vi "Open Baseline Image.vi"(8 "error in (no error)":errorcluster) -> (0 "error out":errorcluster, 2 "dup path":path, 3 "Image Out":T1)   [LabVIEW 2011]
uses:
  <vilib>/vision/Image Controls.llb/IMAQ Image.ctl
  <vilib>/Utility/sysdir.llb/System Directory Type.ctl
  DepthSense/IT WORKS SO SUCK IT/DepthSense Global Status.vi
  <vilib>/vision/NI_Vision_Development_Module.lvlib
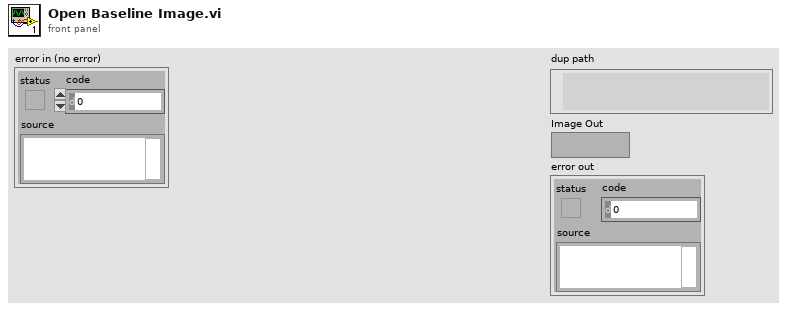
[diagram p1: front panel]
types:
  T1 = typedef "IMAQ Image.ctl" = refnum<image>
  T2 = typedef "System Directory Type.ctl" = i32
  T3 = cluster{"Camera Version":string, "Image Height":i32, "Image Width":i32, "Minimum Framerate":i32, "Maximum Framerate":i32, "Framerate":i32, "Close Mode":bool, "Denoising":bool, "Leakage Algorithm":bool, "Anti-Aliasing":bool, "Camera Status":i32, "API Version":string, "Light Intensity":i32, "Confidence Threshold":u16, "Range":sgl}
  T4 = typedef "Image Type" = u32
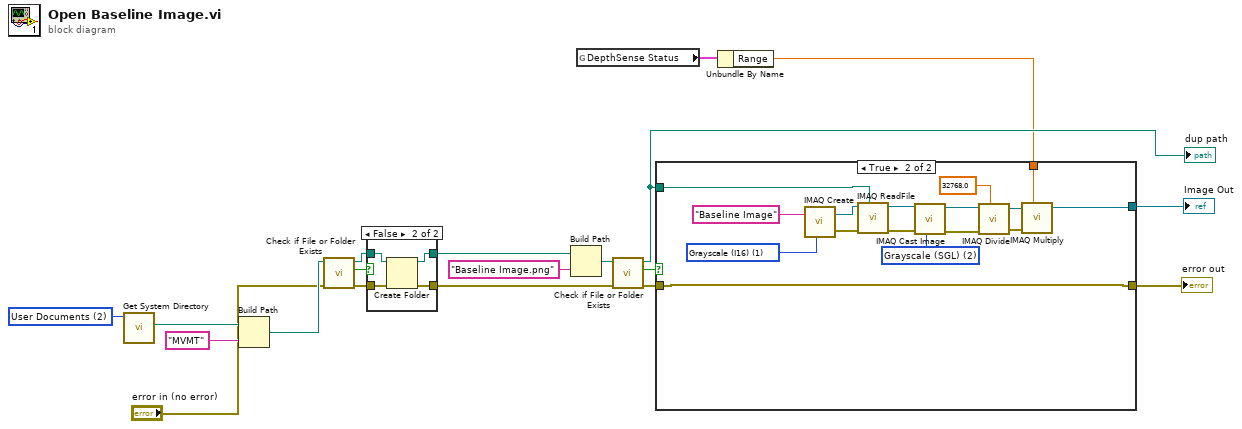
[diagram p0: block diagram]
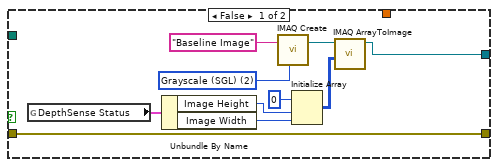
[diagram p2: hidden frame]
diagram:
  w8 = T2 2 items=["User Home"=0, "User Desktop"=1, "User Documents"=2, "User Application Data"=3, "User Preferences"=4, "User Temporary"=5, "Public Documents"=6, "Public Application Data"=7, "Public Preferences"=8, "Public Cache"=13, "System Core Libraries"=9, "System Installed Libraries"=10, "Application Files"=11, "Boot Volume Root"=12] ("system directory type")
  n1 = call <vilib>:"Get System Directory.vi"("system directory type"=w8) -> ("system directory"=w7:path)  [unwired: 10 in]
  n2 = Build Path(base path=w7, name or relative path="MVMT") -> (appended path=w16:path)
  n3 = call <vilib>:"Check if File or Folder Exists.vi"("error in (no error)"="error in (no error)", "path"=w16) -> ("error out"=w17:errorcluster, "file or folder exists?"=w19:bool, "dup path"=w18:path)  [unwired: 7 in]
  n4 = case shown="False" w19 {
    tunnel: w18 -> [w20 w25]
    tunnel: w17 -> [w21 w24]
    tunnel: [w20 w23] -> w14
    tunnel: [w21 w22] -> w11
    frame True {
    }
    frame False {
      n5 = Create Folder(path (use dialog)=w25, error in=w24) -> (created path=w23:path, error out=w22:errorcluster)  [unwired: 1 in, 1 out]
    }
  }
  n6 = Build Path(base path=w14, name or relative path="Baseline Image.png") -> (appended path=w12:path)
  n7 = global read "DepthSense Global Status.vi" "DepthSense Status"() -> (w2:T3)
  n8 = call <vilib>:"Check if File or Folder Exists.vi"("error in (no error)"=w11, "path"=w12) -> ("error out"=w9:errorcluster, "file or folder exists?"=w10:bool, "dup path"=w6:path)  [unwired: 7 in]
  "dup path" <- w6
  n9 = Unbundle By Name(w2) -> ("Range"=w1:sgl)
  n10 = case shown="True" w10 {
    tunnel: w9 -> [w35 w51]
    tunnel: [w35 w51] -> w4
    tunnel: [w26 w36] -> w5
    tunnel: w6 -> [_ w50]
    tunnel: w1 -> [_ w37]
    frame False {
      w28 = T4 2 items=["Grayscale (U8)", "Grayscale (I16)", "Grayscale (SGL)", "Complex (CSG)", "RGB (U32)", "HSL (U32)", "RGB (U64)", "Grayscale (U16)"] ("Image Type")
      n11 = global read "DepthSense Global Status.vi" "DepthSense Status"() -> (w34:T3)
      n12 = Unbundle By Name(w34) -> ("Image Height"=w32:i32, "Image Width"=w31:i32)
      n13 = call "IMAQ Create"("Image Name"="Baseline Image", "Image Type"=w28) -> ("New Image"=w29:T1)  [unwired: 3 in, 1 out]
      n14 = Initialize Array(i16 0, w32, w31) -> (w30:i16[][])
      n15 = call "IMAQ ArrayToImage"("Image Pixels (I16)"=w30, "Image"=w29) -> ("Image Out"=w26:T1)  [unwired: 8 in, 1 out]
    }
    frame True {
      w43 = T4 2 items=["Grayscale (U8)", "Grayscale (I16)", "Grayscale (SGL)", "Complex (CSG)", "RGB (U32)", "HSL (U32)", "RGB (U64)", "Grayscale (U16)"] ("Image Type")
      w46 = T4 1 items=["Grayscale (U8)", "Grayscale (I16)", "Grayscale (SGL)", "Complex (CSG)", "RGB (U32)", "HSL (U32)", "RGB (U64)", "Grayscale (U16)"] ("Image Type")
      n16 = call "IMAQ Create"("Image Name"="Baseline Image", "Image Type"=w46) -> ("New Image"=w49:T1, "error out"=w48:errorcluster)  [unwired: 3 in]
      n17 = call "IMAQ ReadFile"("File Path"=w50, "error in (no error)"=w48, "Image"=w49) -> ("error out"=w45:errorcluster, "Image Out"=w44:T1)  [unwired: 4 in, 3 out]
      n18 = call "IMAQ Cast Image"("Image Type"=w43, "error in (no error)"=w45, "Image Src"=w44) -> ("error out"=w42:errorcluster, "Image Dst Out"=w41:T1)  [unwired: 7 in]
      n19 = call "IMAQ Divide"("Image Src A"=w41, "Constant"=sgl 32768.0, "error in (no error)"=w42) -> ("Image Dst Out"=w39:T1, "error out"=w38:errorcluster)  [unwired: 4 in]
      n20 = call "IMAQ Multiply"("Image Src A"=w39, "Constant"=w37, "error in (no error)"=w38) -> ("Image Dst Out"=w36:T1)  [unwired: 4 in, 1 out]
    }
  }
  "Image Out" <- w5
  "error out" <- w4
